vi "SPIOSet.vi"(4 "DQ(0~15)1":i32=3, 6 "DQ0(0~15)":i32=2, 8 "error in (no error)":errorcluster caption="错误输入（无错误）", 9 "Clock IO(0~15)":i32=1, 10 "CSIO(0~15)":i32, 11 "handle":u64) -> (0 "error out":errorcluster caption="错误输出", 2 "function return":i32, 3 "handle out":u64)   [LabVIEW 2018]
doc: "Set pos. or neg. Supply voltage"
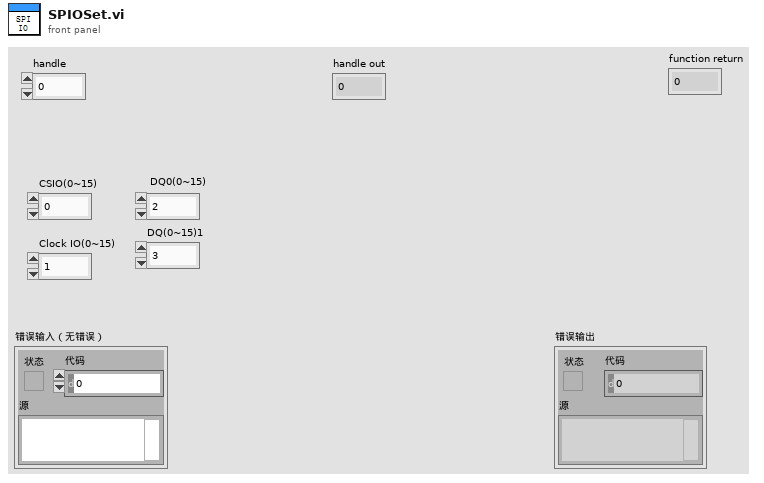
[diagram p1: front panel]
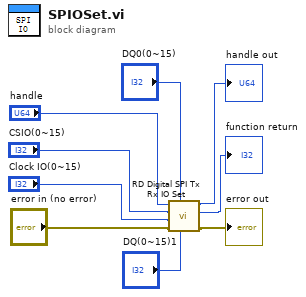
[diagram p0: block diagram]
diagram:
  n1 = call "RD Digital SPI Tx Rx IO Set.vi"("DQ1"="DQ(0~15)1", "DQ0"="DQ0(0~15)", "error in (no error)"="error in (no error)", "ClockDIO"="Clock IO(0~15)", "CSDIO"="CSIO(0~15)", "handle"="handle") -> ("error out"=→"error out":errorcluster, "function return"=→"function return":i32, "handle out"=→"handle out":u64)  [unwired: 3 in]
